vi "Save Current Value as Default.vi"(8 "error in (no error)":errorcluster, 11 "subvi path":path) -> (0 "error out":errorcluster)   [LabVIEW 2018]
panel:
  # "Overview: To Restore the Default Value of the Called VI\nRequirement: LabVIEW Full Development System\nSteps:\n1. Define the directory of the subVI path\n2. Run the VI to restore the default value of the VI"
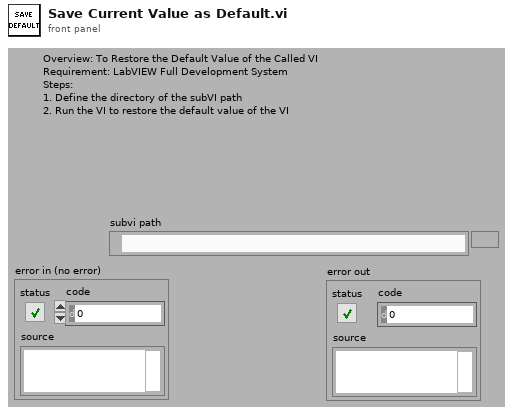
[diagram p1: front panel]
types:
  T1 = enum32{"invalid lock state", "Not Locked", "Locked (No Password)", "Password-protected"}
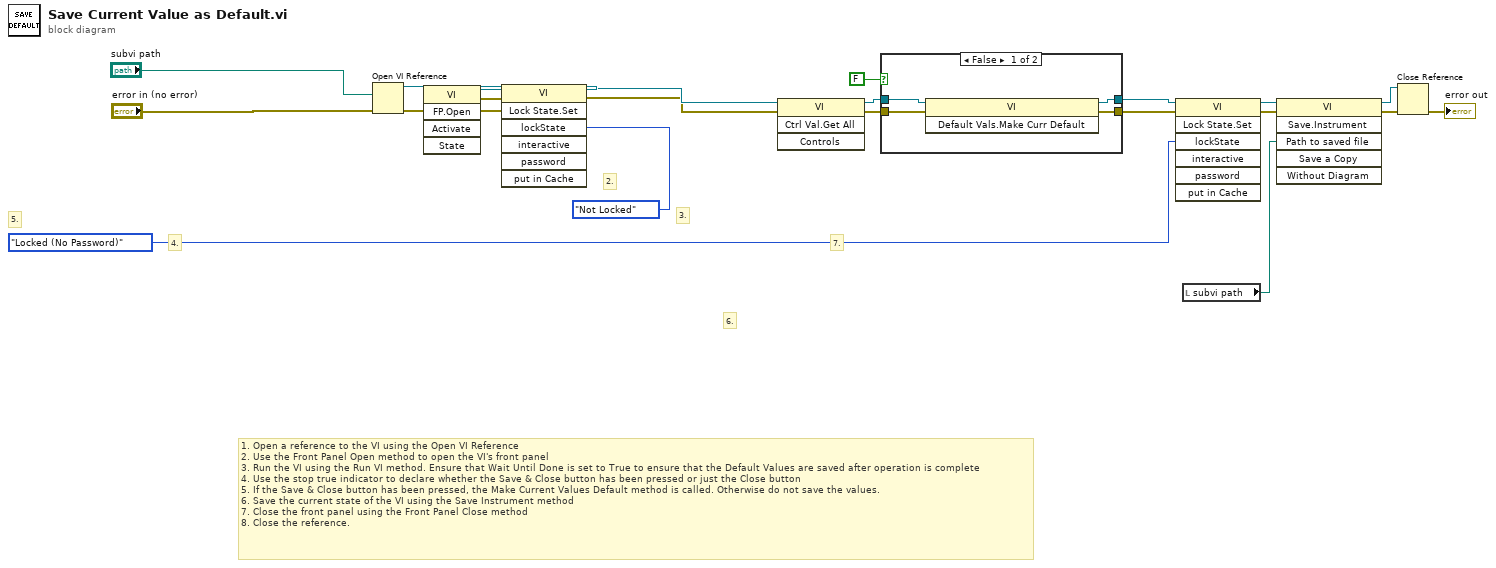
[diagram p0: block diagram]
diagram:
  # "1. Open a reference to the VI using the Open VI Reference\n2. Use the Front Panel Open method to open the VI's front panel\n3. Run the VI using the Run VI method. Ensure that Wait Until Done is set to True to ensure that the Default Values are saved after operation is complete\n4. Use the stop true indicator to declare whether the Save & Close button has been pressed or just the Close button\n5. If the Save & Close button has been pressed, the Make Current Values Default method is called. Otherwise do not save the values.\n6. Save the current state of the VI using the Save Instrument method\n7. Close the front panel using the Front Panel Close method\n8. Close the reference."
  # "7."
  # "6."
  # "5."
  # "4."
  # "3."
  # "2."
  n1 = Open VI Reference(vi path="subvi path", error in (no error)="error in (no error)") -> (vi reference=w21:refnum<vi>, error out=w20:errorcluster)  [unwired: 4 in]
  n2 = invoke class="VI" method="FP.Open"(reference=w21, error in=w20) -> (reference out=w11:refnum<vi>, error out=w10:errorcluster)  [unwired: 3 in, 3 out]
  n3 = invoke class="VI" method="Lock State.Set"(reference=w11, error in=w10, "lockState"=T1."Not Locked" ("Lock State")) -> (reference out=w9:refnum<vi>, error out=w8:errorcluster)  [unwired: 4 in, 5 out]
  n4 = invoke class="VI" method="Ctrl Val.Get All"(reference=w9, error in=w8) -> (reference out=w18:refnum<vi>, error out=w16:errorcluster)  [unwired: 2 in, 2 out]
  n5 = case shown="False" FALSE {
    tunnel: w16 -> [w24 w26]
    tunnel: w18 -> [w25 w27]
    tunnel: [w23 w26] -> w4
    tunnel: [w22 w27] -> w5
    frame False {
      n6 = invoke class="VI" method="Default Vals.Make Curr Default"(reference=w25, error in=w24) -> (reference out=w22:refnum<vi>, error out=w23:errorcluster)  [unwired: 1 in, 1 out]
    }
    frame True {
    }
  }
  n7 = invoke class="VI" method="Lock State.Set"(reference=w5, error in=w4, "lockState"=T1."Locked (No Password)" ("Lock State")) -> (reference out=w6:refnum<vi>, error out=w3:errorcluster)  [unwired: 4 in, 5 out]
  n8 = local read "subvi path"() -> (w12:path)
  n9 = invoke class="VI" method="Save.Instrument"(reference=w6, error in=w3, "Path to saved file"=w12) -> (reference out=w14:refnum<vi>, error out=w13:errorcluster)  [unwired: 3 in, 4 out]
  n10 = Close Reference(reference=w14, error in (no error)=w13) -> (error out=→"error out":errorcluster)
